vi "Post-Build Action.vi"(5 "Files Generated by Build":path[](array[path]), 6 "Top Level/Always Included VIs":path[](array[path]), 7 "Destination Path":path, 8 "error in (no error)":errorcluster, 9 "Target Name":string, 10 "Build Specification Name":string, 11 "Project Path":path) -> (0 "error out":errorcluster)   [LabVIEW 2019]
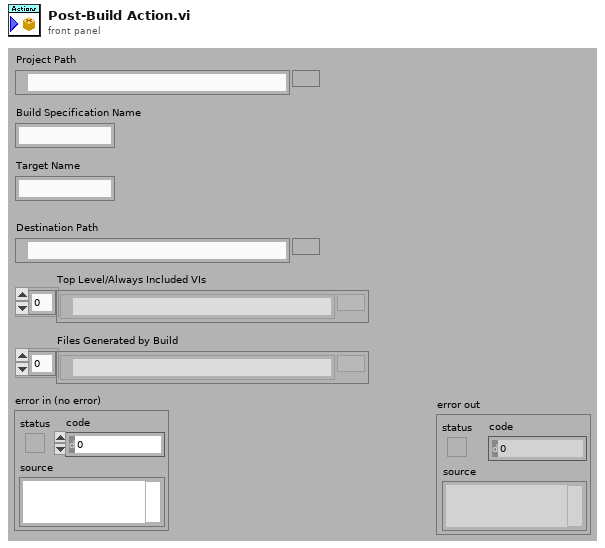
[diagram p1: front panel]
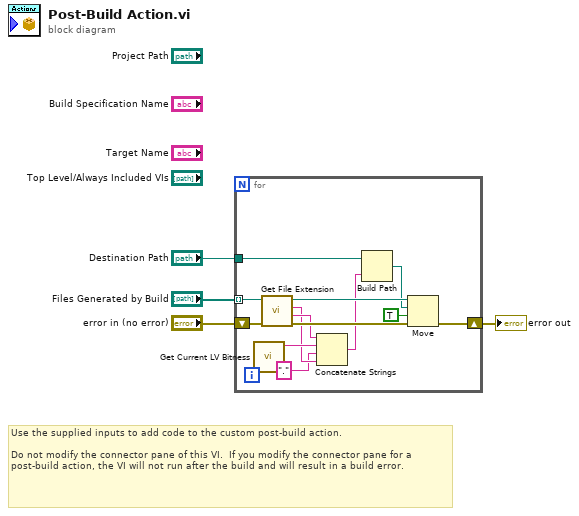
[diagram p0: block diagram]
diagram:
  # "Use the supplied inputs to add code to the custom post-build action.\n\nDo not modify the connector pane of this VI.  If you modify the connector pane for a post-build action, the VI will not run after the build and will result in a build error."
  n1 = for {
    tunnel: "Files Generated by Build" -> [w14] mode=indexing
    shift-right: [w17] -> w2
    shift-left: "error in (no error)" -> [w16]
    tunnel: "Destination Path" -> [w9]
    n2 = call <vilib>:"Get Current LV Bitness.vi"() -> ("bitness"=w12:string)  [unwired: 11 in]
    n3 = call <vilib>:"Get File Extension.vi"("error in (no error)"=w16, "file"=w14) -> ("error out"=w15:errorcluster, "filename without extension"=w13:string, "lowercase file extension"=w11:string, "dup file"=w10:path)  [unwired: 5 in, 1 out]
    n4 = Concatenate Strings(w13, w12, "." ("string"), w11) -> (w8:string)
    n5 = Build Path(base path=w9, name or relative path=w8) -> (appended path=w7:path)
    n6 = Move(source path=w10, error in=w15, 9:TRUE ("overwrite (F)"), 10:w7) -> (error out=w17:errorcluster)  [unwired: 1 in, 2 out]
  }
  "error out" <- w2
